vi "ByteArray2Int.vi"(9 "index":i32, 11 "unsigned byte array":u8[](array[numeric])) -> (3 "number":u32)   [LabVIEW 2012]
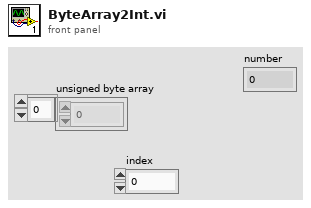
[diagram p1: front panel]
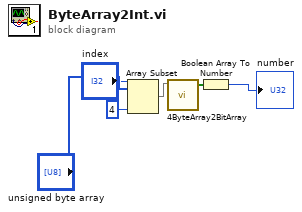
[diagram p0: block diagram]
diagram:
  n1 = Array Subset(array="unsigned byte array", index="index", length=4) -> (w4:u8[])
  n2 = call "4ByteArray2BitArray.vi"("array"=w4) -> ("Array"=w5:bool[])  [unwired: 10 in]
  n3 = Boolean Array To Number(Boolean array=w5) -> (number=→"number":u32)
